vi "Save Crash Log.vi"(6 "error in":errorcluster, 9 "File IO Data":T1={"Work Order Folder"=path "", "Runcount File"=path "", "Report Template Folder"=path "", "Report Folder"=path "", "Report File"=path "", "APU Setup Folder"=path "", "Testing State"=FALSE, "Recording State"=FALSE, "TDMS File Ref"=refnum, "APU Setup File Ref"=refnum, "APU Select"="<Select>", "Test Information"={"APU Part Number:"="", "Model:"="", "Serial Number:"="", "Customer:"="", "Work Order:"="", "Repair Level:"="", "Pre or Post SB"=""}, "Crash Log Data"=[], "Group Name"="", "APU Setup File"={"Sensor Info"=[], "Calibration Info"=[], "CMM Table 106"=[], "CMM Table 106B "=[], "Accel Config"=[], "Report Sheet 1"=[], "Report Sheet 2"=[], "Report Sheet 3"=[]}, "APURunCount"=0}) -> (0 "error out":errorcluster)   [LabVIEW 2018]
doc: "Create file for crash log and write the data in it."
uses:
  File IO.lvlib
  Controller (Host)/Public Controls/Test Information.ctl
  Controller (Host)/Controller (Host).lvlib
  Top Level/Shared Controls/Calculated Data.ctl
  Top Level/Shared Controls/Acq Data.ctl
  Controller (Host)/Public Controls/APU Select.ctl
  Private Controls/File IO Data.ctl
  Top Level/Shared Controls/All Data Cluster.ctl
  Top Level/Shared Controls/Analyzed Data Sets.ctl
  Top Level/Shared Controls/APU Setup File.ctl
panel:
  # "Test Information:"
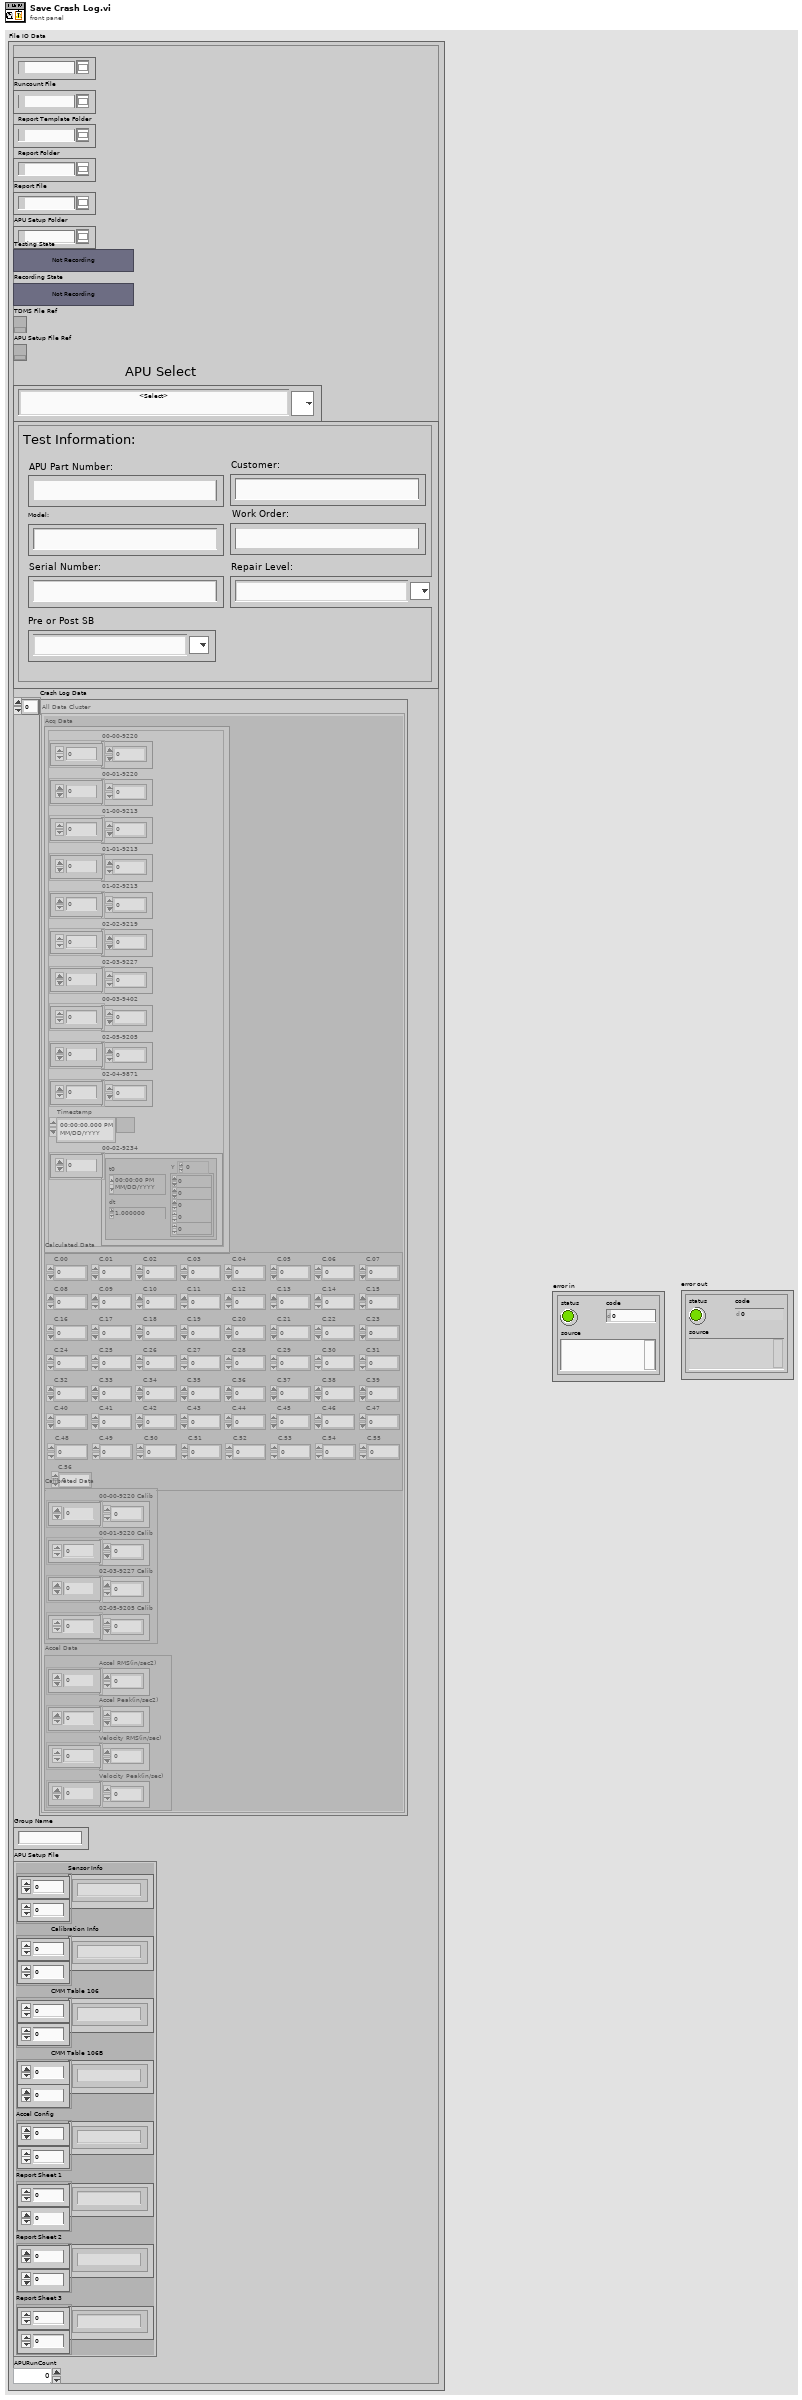
[diagram p1: front panel]
types:
  T1 = typedef "File IO.lvlib/File IO Data.ctl" = cluster{"Work Order Folder":path, "Runcount File":path, "Report Template Folder":path, "Report Folder":path, "Report File":path, "APU Setup Folder":path, "Testing State":bool, "Recording State":bool, "TDMS File Ref":refnum<k34>, "APU Setup File Ref":refnum<k34>, "APU Select":T2, "Test Information":T3, "Crash Log Data":T4, "Group Name":string, "APU Setup File":T8, "APURunCount":u32}
  T2 = typedef "Controller (Host).lvlib/APU Select.ctl" = string
  T3 = typedef "Controller (Host).lvlib/Test Information.ctl" = cluster{"APU Part Number:":string, "Model:":string, "Serial Number:":string, "Customer:":string, "Work Order:":string, "Repair Level:":string, "Pre or Post SB":string}
  T4 = typedef "Analyzed Data Sets.ctl" = T5[]
  T5 = typedef "All Data Cluster.ctl" = cluster{"Acq Data":T6, "Calculated Data":T7, "Calibrated Data":cluster{"00-00-9220 Calib":dbl[], "00-01-9220 Calib":dbl[], "02-03-9227 Calib":dbl[], "02-05-9205 Calib":dbl[]}, "Accel Data":cluster{"Accel RMS(in/sec2)":dbl[], "Accel Peak(in/sec2)":dbl[], "Velocity RMS(in/sec)":dbl[], "Velocity Peak(in/sec)":dbl[]}}
  T6 = typedef "Acq Data.ctl" = cluster{"00-00-9220":dbl[], "00-01-9220":dbl[], "01-00-9213":dbl[], "01-01-9213":dbl[], "01-02-9213":dbl[], "02-02-9219":dbl[], "02-03-9227":dbl[], "00-03-9402":dbl[], "02-05-9205":dbl[], "02-04-9871":dbl[], "Timestamp":timestamp, "00-02-9234":waveform(sgl)[]}
  T7 = typedef "Calculated Data.ctl" = cluster{"C.00":dbl, "C.01":dbl, "C.02":dbl, "C.03":dbl, "C.04":dbl, "C.05":dbl, "C.06":dbl, "C.07":dbl, "C.08":dbl, "C.09":dbl, "C.10":dbl, "C.11":dbl, "C.12":dbl, "C.13":dbl, "C.14":dbl, "C.15":dbl, "C.16":dbl, "C.17":dbl, "C.18":dbl, "C.19":dbl, "C.20":dbl, "C.21":dbl, "C.22":dbl, "C.23":dbl, "C.24":dbl, "C.25":dbl, "C.26":dbl, "C.27":dbl, "C.28":dbl, "C.29":dbl, "C.30":dbl, "C.31":dbl, "C.32":dbl, "C.33":dbl, "C.34":dbl, "C.35":dbl, "C.36":dbl, "C.37":dbl, "C.38":dbl, "C.39":dbl, "C.40":dbl, "C.41":dbl, "C.42":dbl, "C.43":dbl, "C.44":dbl, "C.45":dbl, "C.46":dbl, "C.47":dbl, "C.48":dbl, "C.49":dbl, "C.50":dbl, "C.51":dbl, "C.52":dbl, "C.53":dbl, "C.54":dbl, "C.55":dbl, "C.56":dbl}
  T8 = typedef "APU Setup File.ctl" = cluster{"Sensor Info":string[][], "Calibration Info":string[][], "CMM Table 106":string[][], "CMM Table 106B ":string[][], "Accel Config":string[][], "Report Sheet 1":string[][], "Report Sheet 2":string[][], "Report Sheet 3":string[][]}
  T9 = enum16{"open", "open or create", "create or replace", "create", "open (read-only)"}
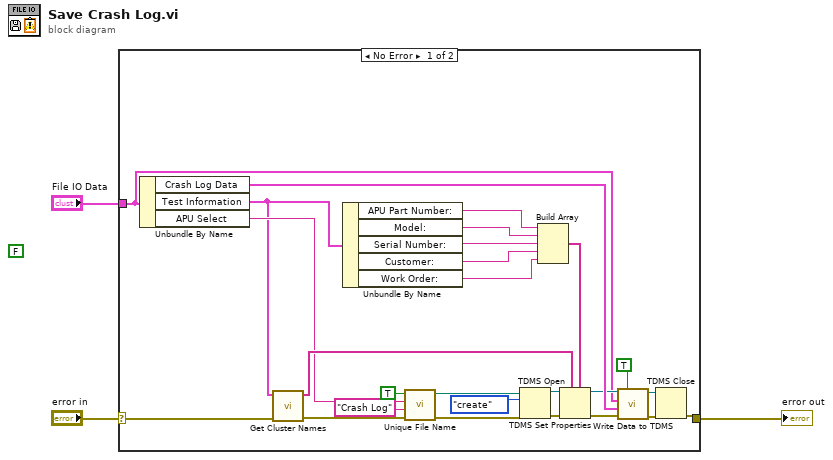
[diagram p0: block diagram]
diagram:
  (unwired) FALSE
  n1 = case shown="No Error" "error in" {
    selector: "error in" -> [w16 w30]
    tunnel: [w11 w30] -> w3
    tunnel: "File IO Data" -> [w4 _]
    frame No Error {
      n2 = Unbundle By Name(w4) -> ("Crash Log Data"=w10:T4, "Test Information"=w12:T3, "APU Select"=w13:T2)
      n3 = call "Get Cluster Names.vi"("error in"=w16, "Test Information"=w12) -> ("error out"=w15:errorcluster, "Cluster Names"=w14:string[])  [unwired: 8 in]
      n4 = Unbundle By Name(w12) -> ("APU Part Number:"=w22:string, "Model:"=w21:string, "Serial Number:"=w20:string, "Customer:"=w19:string, "Work Order:"=w18:string)
      n5 = call "Unique File Name.vi"("error in"=w15, "Folder Name"="Crash Log", "APU Select"=w13, "Crash Log?"=TRUE) -> ("error out"=w26:errorcluster, "Unique File Path"=w25:path)  [unwired: 5 in, 1 out]
      n6 = TDMS Open(8:w26, 10:T9."create" ("operation (0:open)"), 11:w25) -> (0:w28:errorcluster, 3:w29:refnum<k34>)  [unwired: 4 in]
      n7 = Build Array(w22, w21, w20, w19, w18) -> (w17:string[])
      n8 = TDMS Set Properties(5:w17, 7:w14, 8:w28, 11:w29) -> (0:w9:errorcluster, 3:w6:refnum<k34>)  [unwired: 2 in, 2 out]
      n9 = call "Write Data to TDMS.vi"("Crash Log (T)"=TRUE, "error in"=w9, "Data"=w10, "File IO Data In"=w4, "Save Data File Ref In"=w6) -> ("error out"=w8:errorcluster, "Save Data File Ref Out"=w7:refnum<k34>)  [unwired: 4 in, 1 out]
      n10 = TDMS Close(8:w8, 11:w7) -> (0:w11:errorcluster)  [unwired: 1 out]
    }
    frame Error {
    }
  }
  "error out" <- w3
